vi "Get Time Alarm Str V.vi"(8 "error in (no error)":errorcluster) -> (0 "error out":errorcluster, 3 "function return":string)   [LabVIEW 2009, in "VantagePro.lvlib"]
doc: "DllAccess char* _stdcall GetTimeAlarmStr_V (void);"
uses:
  VantagePro.lvlib
  <userlib>/VantagePro/VantagePro.dll
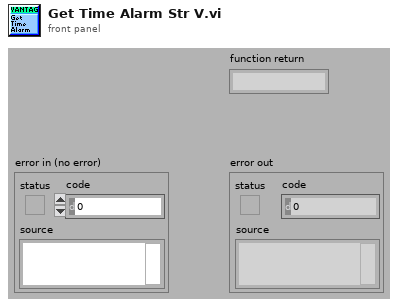
[diagram p1: front panel]
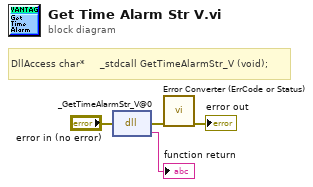
[diagram p0: block diagram]
diagram:
  # "DllAccess char*     _stdcall GetTimeAlarmStr_V (void);"
  n1 = dll-call lib="C:/Program Files/National Instruments/LabVIEW 2010/user.lib/VantagePro/VantagePro.*" fn="_GetTimeAlarmStr_V@0"(error in="error in (no error)") -> (error out=w2:errorcluster, →"function return":string)  [unwired: 2 in, 1 out]
  n2 = call "Error Converter (ErrCode or Status).vi"("error in (no error)"=w2) -> ("error out"=→"error out":errorcluster)  [unwired: 10 in]
